vi "Read Buckets.vi"(8 "error in (no error)":errorcluster, 11 "Histogram in":refnum<class "Histogram.lvclass">) -> (0 "error out":errorcluster, 2 "Buckets":dbl[](array[numeric]), 3 "Histogram out":refnum<class "Histogram.lvclass">)   [LabVIEW 2020, in "Metrics.lvlib" / "Histogram.lvclass"]
uses:
  Histogram.lvclass
  Histogram.lvclass/Histogram.ctl
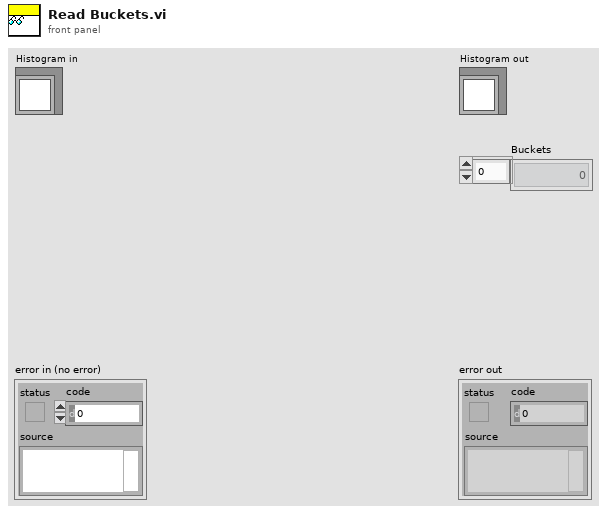
[diagram p1: front panel]
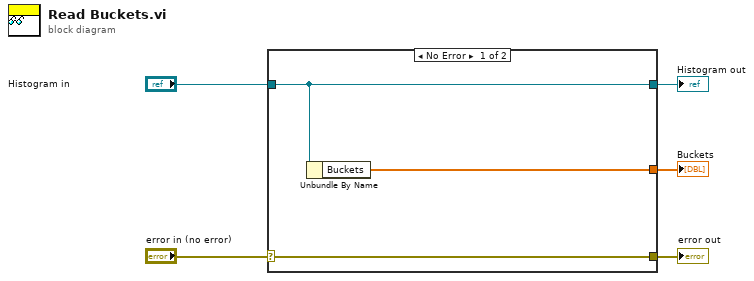
[diagram p0: block diagram]
diagram:
  n1 = case shown="No Error" "error in (no error)" {
    selector: "error in (no error)" -> [w8 w9]
    tunnel: [w8 w9] -> w4
    tunnel: [w7 w10] -> w2
    tunnel: "Histogram in" -> [w7 w10]
    tunnel: [w6 _] -> w1
    frame No Error {
      n2 = Unbundle By Name(w7) -> ("Buckets"=w6:dbl[])
    }
    frame Error {
    }
  }
  "error out" <- w4
  "Histogram out" <- w2
  "Buckets" <- w1
